vi "XYgraph1MOD.vi"() -> ()   [LabVIEW 2021]
panel:
  out "XY Graph":cluster{"X":dbl[], "Y":dbl[]}[](graph)
  in  "stop":bool
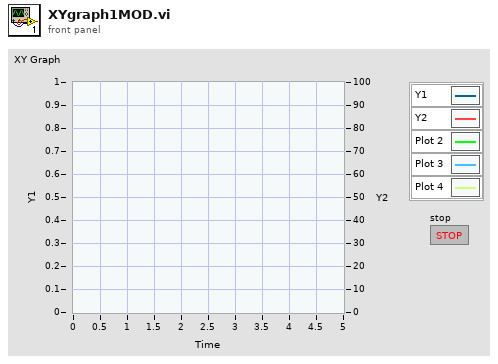
[diagram p1: front panel]
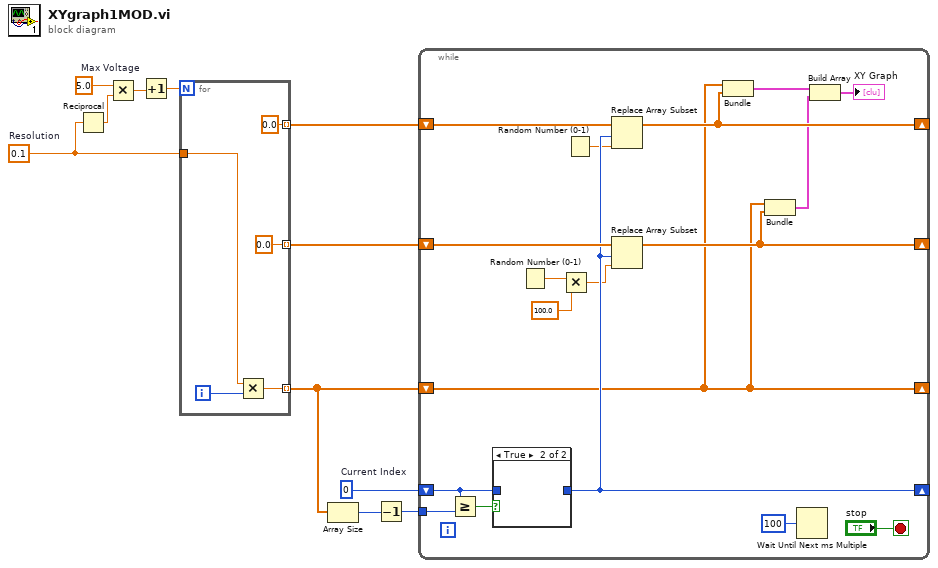
[diagram p0: block diagram]
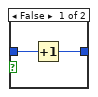
[diagram p2: hidden frame]
diagram:
  w6 = 5.0  # Max Voltage
  w5 = 0.1  # Resolution
  w11 = 0  # Current Index
  n1 = Reciprocal(x=w5) -> (1/x=w7:dbl)
  n2 = Multiply(x=w6, y=w7) -> (x*y=w4:dbl)
  n3 = Increment(x=w4) -> (x+1=w8:dbl)
  n4 = for {
    N: w8 -> [_]
    tunnel: [0.0] -> w2 mode=indexing
    tunnel: w5 -> [w15]
    tunnel: [w13] -> w3 mode=indexing
    tunnel: [0.0] -> w1 mode=indexing
    i -> [w14]
    n5 = Multiply(x=w15, y=w14) -> (x*y=w13:dbl)
  }
  n6 = Array Size(array=w3) -> (size(s)=w10:i32)
  n7 = Decrement(x=w10) -> (x-1=w9:i32)
  n8 = while {
    shift-right: [w25] -> _
    shift-left: w11 -> [w32]
    shift-right: [w23] -> _
    shift-left: w3 -> [w23]
    tunnel: w9 -> [w30]
    shift-right: [w27] -> _
    shift-left: w2 -> [w28]
    shift-right: [w24] -> _
    shift-left: w1 -> [w26]
    stop <- "stop" stop-if-true
    n9 = Greater Or Equal?(x=w32, y=w30) -> (x >= y?=w31:bool)
    n10 = case shown="True" w31 {
      tunnel: w32 -> [w36 _]
      tunnel: [w35 _] -> w25
      frame False {
        n11 = Increment(x=w36) -> (x+1=w35:i32)
      }
      frame True {
      }
    }
    n12 = Random Number (0-1)() -> (number: 0 to 1=w19:dbl)
    n13 = Multiply(x=w19, y=100.0) -> (x*y=w18:dbl)
    n14 = Random Number (0-1)() -> (number: 0 to 1=w20:dbl)
    n15 = Replace Array Subset(array=w26, new element=w20, index=w25) -> (w24:dbl[])
    n16 = Replace Array Subset(array=w28, new element=w18, index=w25) -> (w27:dbl[])
    n17 = Bundle(w23, w24) -> (w22:cluster{dbl[], dbl[]})  [unwired: 1 in]
    n18 = Bundle(w23, w27) -> (w21:cluster{dbl[], dbl[]})  [unwired: 1 in]
    n19 = Wait Until Next ms Multiple(millisecond multiple=u32 100) -> ()  [unwired: 1 out]
    n20 = Build Array(w22, w21) -> (→"XY Graph":cluster{dbl[], dbl[]}[])
  }
